vi "存数据cloumns(子VI).vi"() -> (3 "数组":string[](array[string]))   [LabVIEW 2016, in "斯坦道CODMn.lvlib"]
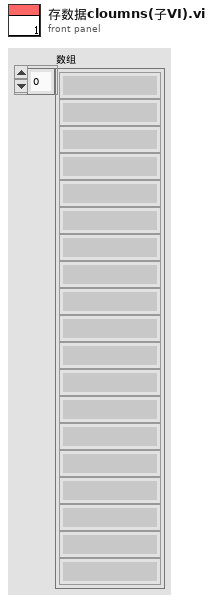
[diagram p1: front panel]
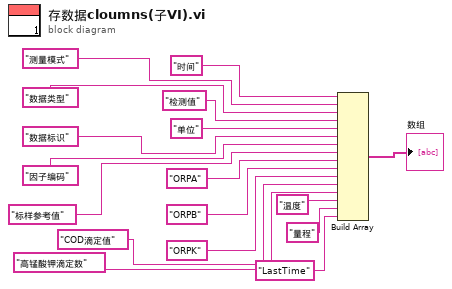
[diagram p0: block diagram]
diagram:
  n1 = Build Array("时间", "测量模式", "数据类型", "检测值", "单位", "数据标识", "因子编码", "标样参考值", "ORPA", "ORPB", "ORPK", "COD滴定值", "高锰酸钾滴定数", "温度", "量程" ("元素"), "LastTime" ("元素")) -> (→"数组":string[])
